vi "Create Tab of FolderFiles.vi"(8 "error in (no error)":errorcluster, 11 "Folder_Mgmt in":refnum<class "Folder_Mgmt.lvclass">) -> (0 "error out":errorcluster, 3 "Folder_Mgmt out":refnum<class "Folder_Mgmt.lvclass">)   [LabVIEW 2016, in "Folder_Mgmt.lvclass"]
uses:
  Folder_Mgmt.lvclass
  Folder_Mgmt.lvclass/Folder_Mgmt.ctl
  <userlib>/_OpenG.lib/array/array.llb/Delete Elements from 1D Array (Path)__ogtk.vi
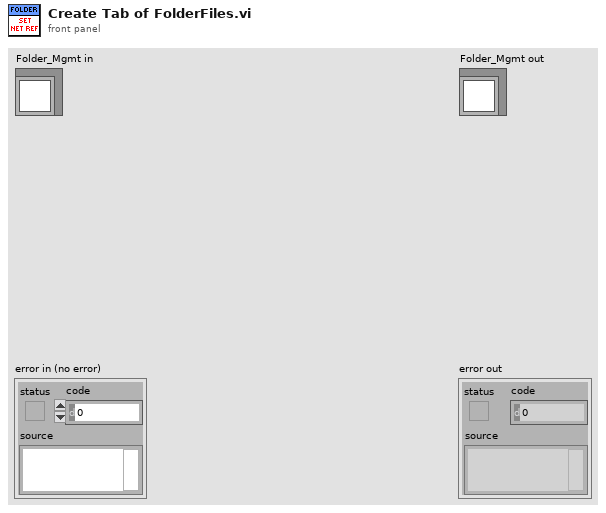
[diagram p1: front panel]
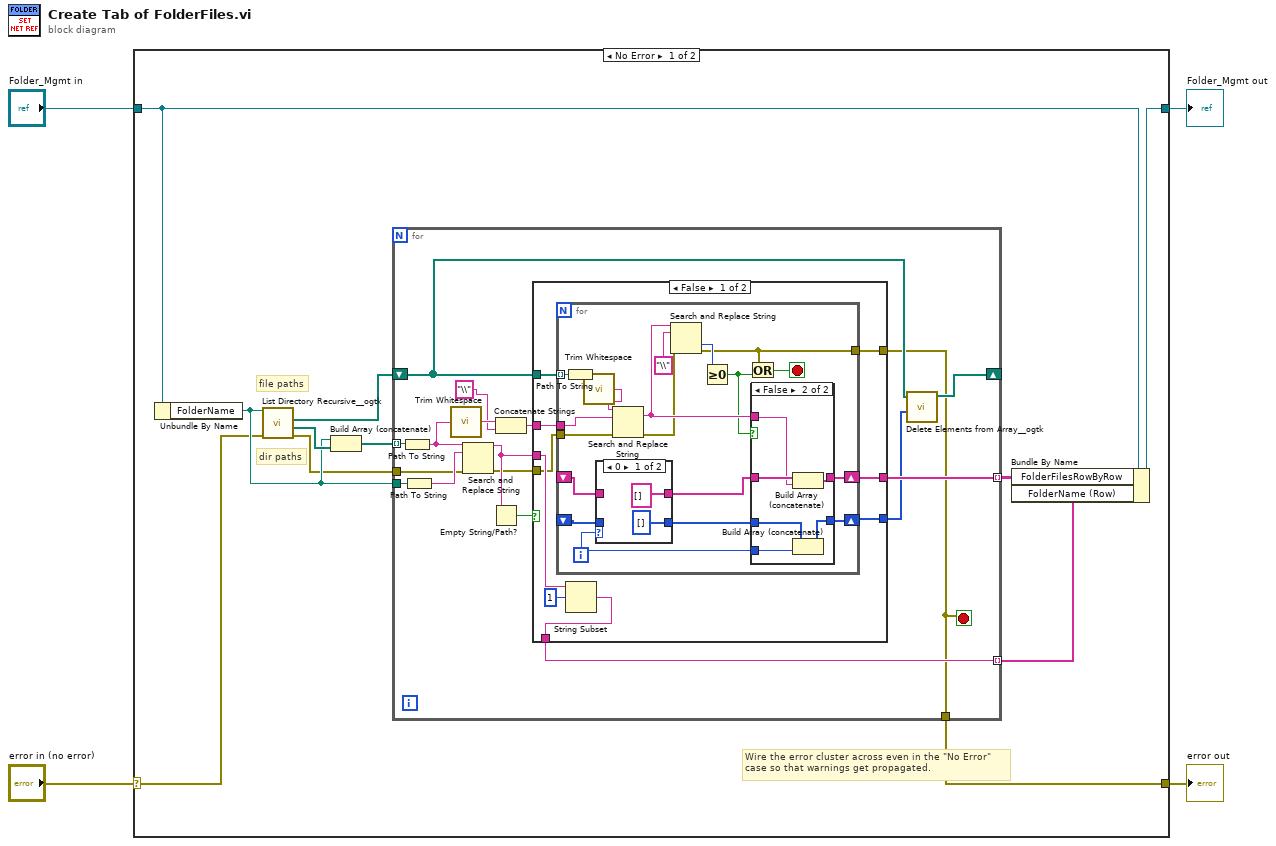
[diagram p0: block diagram]
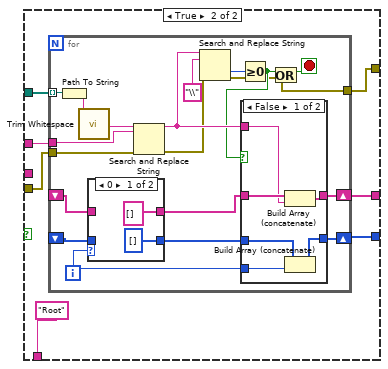
[diagram p4: hidden frame]
diagram:
  n1 = case shown="No Error" "error in (no error)" {
    selector: "error in (no error)" -> [w6 w112]
    tunnel: [w5 w112] -> w3
    tunnel: [w14 w111] -> w1
    tunnel: "Folder_Mgmt in" -> [w15 w111]
    frame No Error {
      # "dir paths"
      # "file paths"
      # "Wire the error cluster across even in the \"No Error\"\ncase so that warnings get propagated."
      n2 = Unbundle By Name(w15) -> ("FolderName"=w10:path)
      n3 = call <userlib>:"List Directory Recursive__ogtk.vi"("error in (no error)"=w6, "Path"=w10) -> ("error out"=w7:errorcluster, "dir paths"=w13:path[], "file paths"=w12:path[])  [unwired: 6 in, 1 out]
      n4 = Build Array (concatenate)(w10, w13) -> (w11:path[])
      n5 = for {
        tunnel: w11 -> [w31] mode=indexing
        tunnel: [w32] -> w9 mode=indexing
        shift-right: [w29] -> _
        shift-left: w12 -> [w25]
        tunnel: w10 -> [w28]
        tunnel: [w26] -> w8 mode=indexing
        tunnel: w7 -> [w18]
        tunnel: [w16] -> w5
        stop <- w16 stop-if-true
        n6 = Path To String(path=w31) -> (string=w19:string)
        n7 = Path To String(path=w28) -> (string=w24:string)
        n8 = call <vilib>:"Trim Whitespace.vi"("string"=w19) -> ("trimmed string"=w22:string)  [unwired: 1 in]
        n9 = Search and Replace String(input string=w19, search string=w24, error in=w18) -> (result string=w23:string, error out=w17:errorcluster)  [unwired: 5 in, 2 out]
        n10 = Empty String/Path?(string/path=w23) -> (empty?=w27:bool)
        n11 = Concatenate Strings(w22, "\\" ("regular expression")) -> (w20:string)
        n12 = case shown="False" w27 {
          tunnel: [w41 w79] -> w32
          tunnel: [w40 w78] -> w30
          tunnel: w25 -> [w39 w77]
          tunnel: w23 -> [w37 _]
          tunnel: [w35 "Root"] -> w26
          tunnel: w20 -> [w38 w75]
          tunnel: w17 -> [w34 w74]
          tunnel: [w33 w73] -> w16
          frame False {
            n13 = for {
              tunnel: w39 -> [w60] mode=indexing
              shift-right: [w59] -> w41
              shift-left: _ -> [w58]
              shift-right: [w54] -> w40
              shift-left: _ -> [w53]
              tunnel: w38 -> [w46]
              tunnel: w34 -> [w45]
              tunnel: [w42] -> w33
              i -> [w56]
              stop <- w43 stop-if-true
              n14 = Path To String(path=w60) -> (string=w50:string)
              n15 = call <vilib>:"Trim Whitespace.vi"("string"=w50) -> ("trimmed string"=w47:string)  [unwired: 1 in]
              n16 = case shown="0" w56 {
                tunnel: w58 -> [_ w64]
                tunnel: [string[] [] w64] -> w57
                tunnel: [i32[] [] w63] -> w55
                tunnel: w53 -> [_ w63]
                frame 0 {
                }
                frame 1, Default {
                }
              }
              n17 = Search and Replace String(input string=w47, search string=w46, error in=w45) -> (result string=w49:string, error out=w44:errorcluster)  [unwired: 5 in, 2 out]
              n18 = Search and Replace String(input string=w49, search string="\\" ("regular expression"), error in=w44) -> (offset past replacement=w51:i32, error out=w42:errorcluster)  [unwired: 5 in, 2 out]
              n19 = Greater Or Equal To 0?(x=w51) -> (x >= 0?=w48:bool)
              n20 = Or(x=w42, y=w48) -> (x .or. y?=w43:bool)
              n21 = case shown="False" w48 {
                tunnel: w57 -> [w66 w71]
                tunnel: [w66 w72] -> w59
                tunnel: w49 -> [_ w67]
                tunnel: w56 -> [_ w70]
                tunnel: w55 -> [w65 w69]
                tunnel: [w65 w68] -> w54
                frame True {
                }
                frame False {
                  n22 = Build Array (concatenate)(w71, w67) -> (w72:string[])
                  n23 = Build Array (concatenate)(w69, w70) -> (w68:i32[])
                }
              }
            }
            n24 = String Subset(string=w37, offset (0)=1) -> (substring=w35:string)  [unwired: 1 in]
          }
          frame True {
            n25 = for {
              tunnel: w77 -> [w91] mode=indexing
              shift-right: [w98] -> w79
              shift-left: _ -> [w97]
              shift-right: [w93] -> w78
              shift-left: _ -> [w92]
              tunnel: w75 -> [w84]
              tunnel: w74 -> [w83]
              tunnel: [w80] -> w73
              i -> [w95]
              stop <- w81 stop-if-true
              n26 = Path To String(path=w91) -> (string=w90:string)
              n27 = call <vilib>:"Trim Whitespace.vi"("string"=w90) -> ("trimmed string"=w85:string)  [unwired: 1 in]
              n28 = case shown="0" w95 {
                tunnel: w97 -> [_ w110]
                tunnel: [string[] [] w110] -> w96
                tunnel: [i32[] [] w109] -> w94
                tunnel: w92 -> [_ w109]
                frame 0 {
                }
                frame 1, Default {
                }
              }
              n29 = Search and Replace String(input string=w85, search string=w84, error in=w83) -> (result string=w87:string, error out=w82:errorcluster)  [unwired: 5 in, 2 out]
              n30 = Search and Replace String(input string=w87, search string="\\" ("regular expression"), error in=w82) -> (offset past replacement=w88:i32, error out=w80:errorcluster)  [unwired: 5 in, 2 out]
              n31 = Greater Or Equal To 0?(x=w88) -> (x >= 0?=w86:bool)
              n32 = case shown="False" w86 {
                tunnel: [w104 w106] -> w98
                tunnel: w96 -> [w103 w106]
                tunnel: w95 -> [w102 _]
                tunnel: w94 -> [w101 w105]
                tunnel: [w100 w105] -> w93
                tunnel: w87 -> [w99 _]
                frame False {
                  n33 = Build Array (concatenate)(w103, w99) -> (w104:string[])
                  n34 = Build Array (concatenate)(w101, w102) -> (w100:i32[])
                }
                frame True {
                }
              }
              n35 = Or(x=w86, y=w80) -> (x .or. y?=w81:bool)
            }
          }
        }
        n36 = call-poly <userlib>:"Delete Elements from Array__ogtk.vi"("indices"=w30, "array"=w25) -> ("array w/ subset deleted"=w29:path[])  [unwired: 8 in, 1 out]
      }
      n37 = Bundle By Name(cluster=w15, "FolderFilesRowByRow"=w9, "FolderName (Row)"=w8) -> (w14:refnum<class "Folder_Mgmt.lvclass">)
    }
    frame Error {
    }
  }
  "error out" <- w3
  "Folder_Mgmt out" <- w1
